vi "BRig_Host_comm_tcp_parseCmd__getType_v3.vi"(0 "input_strCmd":string, 2 "input_countCmd":i32) -> (14 "output_strType":u8)   [LabVIEW 2014]
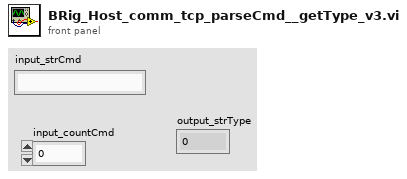
[diagram p1: front panel]
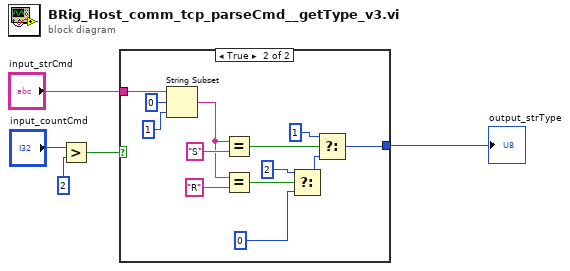
[diagram p0: block diagram]
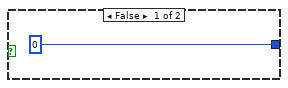
[diagram p2: hidden frame]
diagram:
  n1 = Greater?(x="input_countCmd", y=2) -> (0:w3:bool)
  n2 = case shown="True" w3 {
    tunnel: "input_strCmd" -> [_ w8]
    tunnel: [u8 0 ("t") w13] -> w2
    frame False {
    }
    frame True {
      n3 = String Subset(string=w8, offset (0)=0, length (rest)=1 ("length (rest)")) -> (substring=w9:string)
      n4 = Equal?(x=w9, y="S") -> (x = y?=w10:bool)
      n5 = Equal?(x=w9, y="R") -> (x = y?=w11:bool)
      n6 = Select(t=u8 2, s=w11, f=u8 0) -> (s? t:f=w14:u8)
      n7 = Select(t=u8 1, s=w10, f=w14) -> (s? t:f=w13:u8)
    }
  }
  "output_strType" <- w2
